vi "Build core.vi"(6 "Previous Build's Artifacts":refnum<class "Build Artifact.lvclass">[](array[class]), 7 "Progress":refnum<class "Progress.lvclass">, 8 "error in (no error)":errorcluster, 10 "Build Cache":refnum<class "Build Cache.lvclass">, 11 "Build Item in":refnum<class "Apply VIPC Step.lvclass">) -> (0 "error out":errorcluster, 1 "Explore Path":path, 2 "Build Results":T1, 4 "New Artifacts":refnum<class "Build Artifact.lvclass">[](array[class]))   [LabVIEW 2019, in "VIPM.lvlib" / "Apply VIPC Step.lvclass"]
doc: "Performs all the necessary build actions for the build step.\n\nCopyright: MGI 2016\nAuthor: Derek Trepanier"
uses:
  Apply VIPC Step.lvclass
  C:/Users/pasca/source/repos/mgi-solution-explorer-extensions/libs/Solution.lvlibp/Solution/Build Item/Build Step.lvclass
  libs/Solution.lvlibp/Solution/Progress/Progress.lvclass
  libs/Solution.lvlibp/Solution/Build Artifact/Build Artifact.lvclass
  libs/Solution.lvlibp/Solution/Build Item/Build Result.ctl
  libs/Solution.lvlibp/Solution/Build Cache/Build Cache.lvclass
  Apply VIPC Step.lvclass/Apply VIPC Step.ctl
  libs/Solution.lvlibp/Solution/Build Item/Read LV Year.vi
  libs/Solution.lvlibp/Solution/Build Item/Build Step.lvclass
  <vilib>/JKI/VIPM API/VIPM API_vipm_api.lvlib
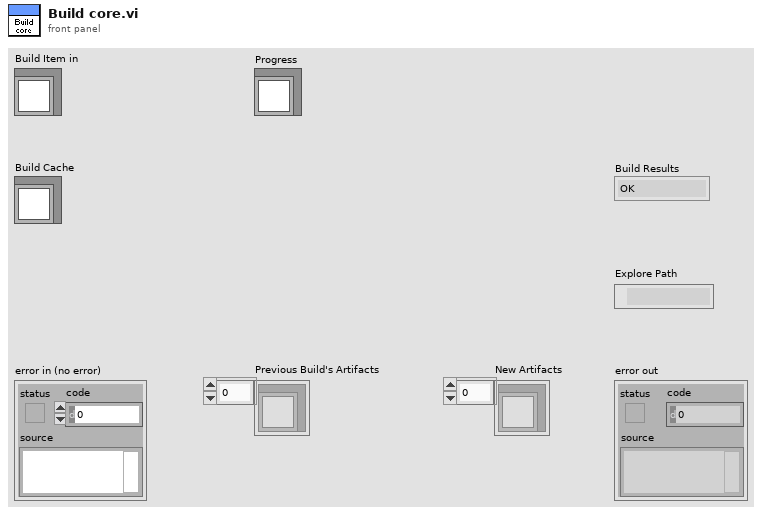
[diagram p1: front panel]
types:
  T1 = typedef "Solution.lvlibp/Build Step.lvclass/Build Result.ctl" = enum16{"OK", "Skipped", "Error"}
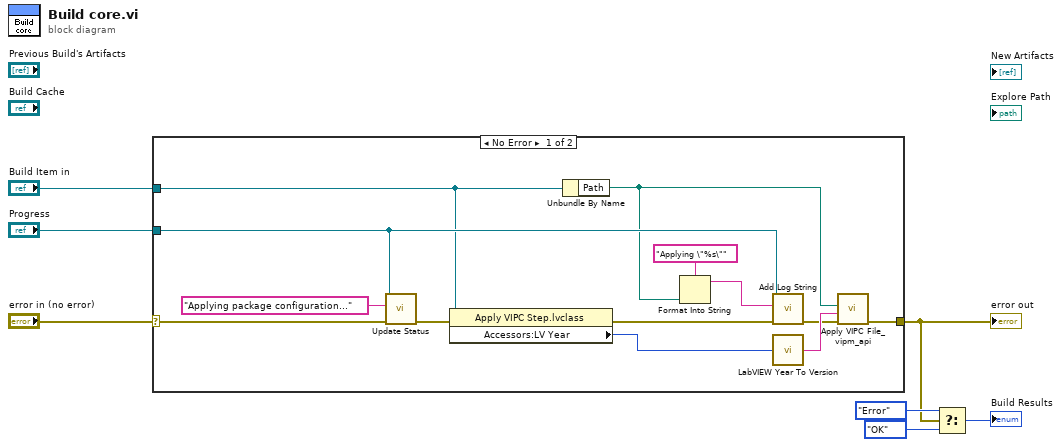
[diagram p0: block diagram]
diagram:
  n1 = case shown="No Error" "error in (no error)" {
    selector: "error in (no error)" -> [w20 w21]
    tunnel: [w15 w21] -> w4
    tunnel: "Build Item in" -> [w13 _]
    tunnel: "Progress" -> [w18 _]
    frame No Error {
      n2 = call "Update Status.vi"("error in (no error)"=w20, "Status String"="Applying package configuration...", "Progress in"=w18) -> ("error out"=w9:errorcluster)  [unwired: 8 in]
      n3 = property class="Apply VIPC Step.lvclass"(reference=w13, error in=w9) -> (error out=w10:errorcluster, "Accessors:LV Year"=w12:u32)  [unwired: 1 out]
      n4 = Unbundle By Name(w13) -> ("Path"=w14:path)
      n5 = Format Into String(format string="Applying \"%s\"" ("Log Item"), w14) -> (resulting string=w17:string)  [unwired: 2 in, 1 out]
      n6 = call "Add Log String.vi"("error in (no error)"=w10, "Log Item"=w17, "Progress in"=w18) -> ("error out"=w8:errorcluster)  [unwired: 8 in]
      n7 = call "LabVIEW Year To Version.vi"("LabVIEW Year"=w12) -> ("LabVIEW Version"=w11:string)  [unwired: 1 in]
      n8 = call <vilib>:"Apply VIPC File_vipm_api.vi"("error in (no error)"=w8, "LabVIEW Version"=w11, "VIPC File"=w14) -> ("error out"=w15:errorcluster)  [unwired: 8 in]
    }
    frame Error {
    }
  }
  "error out" <- w4
  n9 = Select(t=Build_Result."Error" ("Build Results"), s=w4, f=Build_Result."OK" ("Build Results")) -> (s? t:f=→"Build Results":T1)
